vi "Fix Coercion Dots.vi"() -> ()   [LabVIEW 2020]
panel:
  out "Timestamp indicator":timestamp
  out "Complex Answer":cdb
  out "Numeric":i32
  out "x+y":u64
  in  "Offset (I32)":i32
  in  "Scale Factor (DBL)":dbl
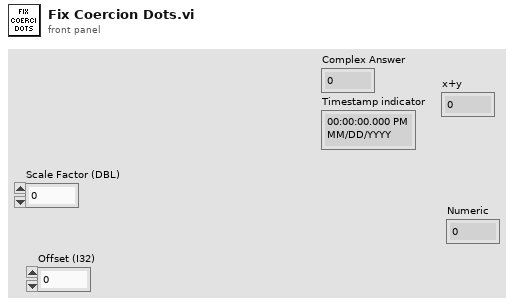
[diagram p1: front panel]
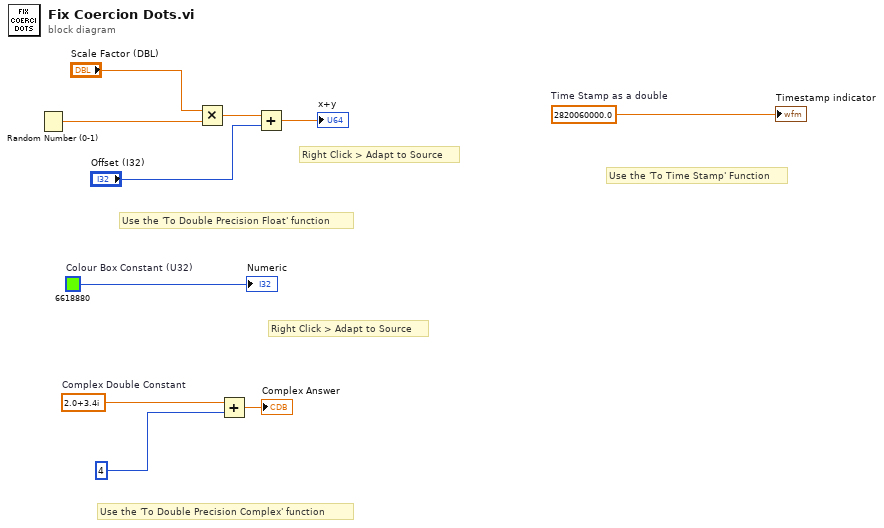
[diagram p0: block diagram]
diagram:
  w1 = 2820060000.0  # Time Stamp as a double
  w4 = cdb 2.0+3.4i  # Complex Double Constant
  w5 = u32 6618880  # Colour Box Constant (U32)
  # "Use the 'To Time Stamp' Function"
  # "Use the 'To Double Precision Complex' function"
  # "Right Click > Adapt to Source"
  # "Use the 'To Double Precision Float' function"
  # "Right Click > Adapt to Source"
  n1 = Random Number (0-1)() -> (number: 0 to 1=w9:dbl)
  n2 = Multiply(x="Scale Factor (DBL)", y=w9) -> (x*y=w8:dbl)
  n3 = Add(x=w4, y=4) -> (x+y=→"Complex Answer":cdb)
  n4 = Add(x=w8, y="Offset (I32)") -> (x+y=→"x+y":dbl)
  "Numeric" <- w5
  "Timestamp indicator" <- w1
